vi "PID test.vi"(8 "Enable PID":bool) -> ()   [LabVIEW 2014]
uses:
  PIDstatemachinectl.ctl
  <vilib>/Rock Robotics/WPI/RobotDrive/WPI_RobotDriveGetSetRefNum.vi
panel:
  in  "PID state machine":T1
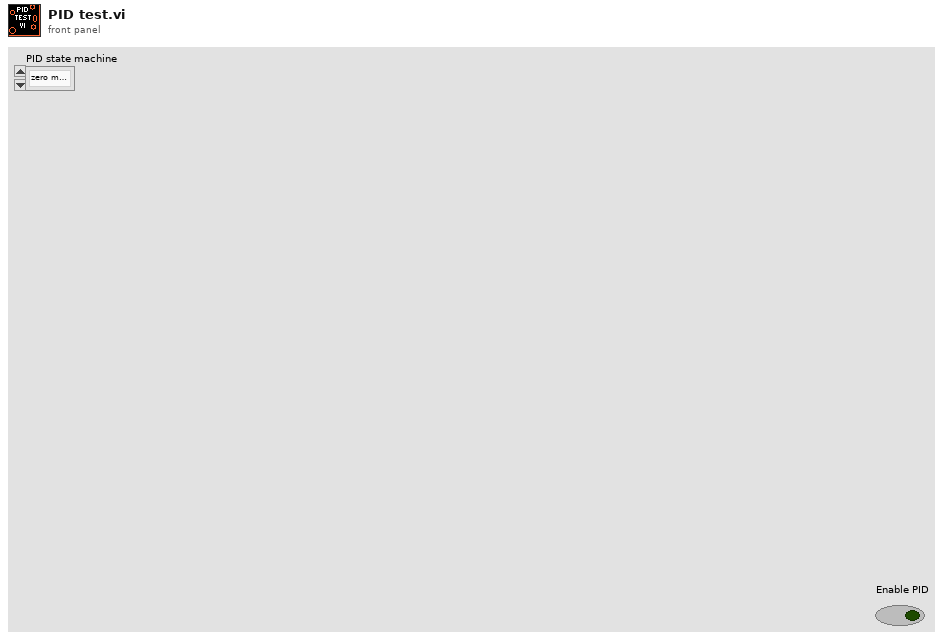
[diagram p1: front panel]
types:
  T1 = typedef "PIDstatemachinectl.ctl" = enum16{"zero motors", "set/run pid", "reset encoder"}
  T2 = typedef "WPI_RobotDriveDevRef.ctl" = cluster{"DevStatus":errorcluster, "Motors[]":T3[], "Square Inputs":bool, "Max Output":dbl}
  T3 = typedef "WPI_MotorControlDeviceRef.ctl" = cluster{"DeviceStatus":errorcluster, "Type":T4, "PWM":cluster{"Controller":T5, "PWM Channel":T6, "DeadBand":T7}, "CAN":cluster{"Device Number":u8, "Control Mode":T8, "Semaphore":T9, "Max Vout":dbl, "TalonSRX Control Mode":T10}, "Invert":bool, "TransformRef":T11, "InvTransformRef":T11}
  T4 = typedef "WPI_MotorControlType.ctl" = enum16{"PWM", "CAN", "CANTalonSRX"}
  T5 = typedef "FPGA_TypedefDigitalModule.ctl" = enum16{"Controller 1"}
  T6 = typedef "FPGA_DIOPWMChannel.ctl" = enum8{"PWM 0", "PWM 1", "PWM 2", "PWM 3", "PWM 4", "PWM 5", "PWM 6", "PWM 7", "PWM 8", "PWM 9", "PWM MXP 0", "PWM MXP 1", "PWM MXP 2", "PWM MXP 3", "PWM MXP 4", "PWM MXP 5", "PWM MXP 6", "PWM MXP 7", "PWM MXP 8", "PWM MXP 9", "Invalid"}
  T7 = typedef "WPI_PWMDeadband.ctl" = cluster{"Name":string, "maxPositivePwm":i32, "minPositivePwm":i32, "centerPwm":i32, "maxNegativePwm":i32, "minNegativePwm":i32, "angularRange":u16}
  T8 = typedef "WPI_CANJaguar_ControlMode.ctl" = enum8{"Percent VBus", "Current", "Speed", "Position", "Voltage"}
  T9 = typedef "Semaphore RefNum" = refnum<k1>
  T10 = typedef "WPI_CANTalonSRX_APIControlMode.ctl" = enum8{"Percent VBus", "Speed", "Position", "Slave", "Unchanged / Invalid"}
  T11 = typedef "WPI_PWMTransform_ConPane.ctl" = refnum<vi>
  T12 = typedef "WPI_EncoderDevRef.ctl" = cluster{"DevStatus":errorcluster, "EncoderIndex":T13, "CounterIndex":T14, "DistancePerCount":dbl, "Decoding Type":T15}
  T13 = typedef "FPGA_EncoderIdx.ctl" = enum8{"Enc 0", "Enc 1", "Enc 2", "Enc 3", "Enc 4", "Enc 5", "Enc 6", "Enc 7", "Invalid"}
  T14 = typedef "FPGA_CounterCtrSystemIndex.ctl" = enum8{"Ctr 0", "Ctr 1", "Ctr 2", "Ctr 3", "Ctr 4", "Ctr 5", "Ctr 6", "Ctr 7", "Invalid"}
  T15 = typedef "WPI_EncoderType.ctl" = enum16{"1x", "2x", "4x"}
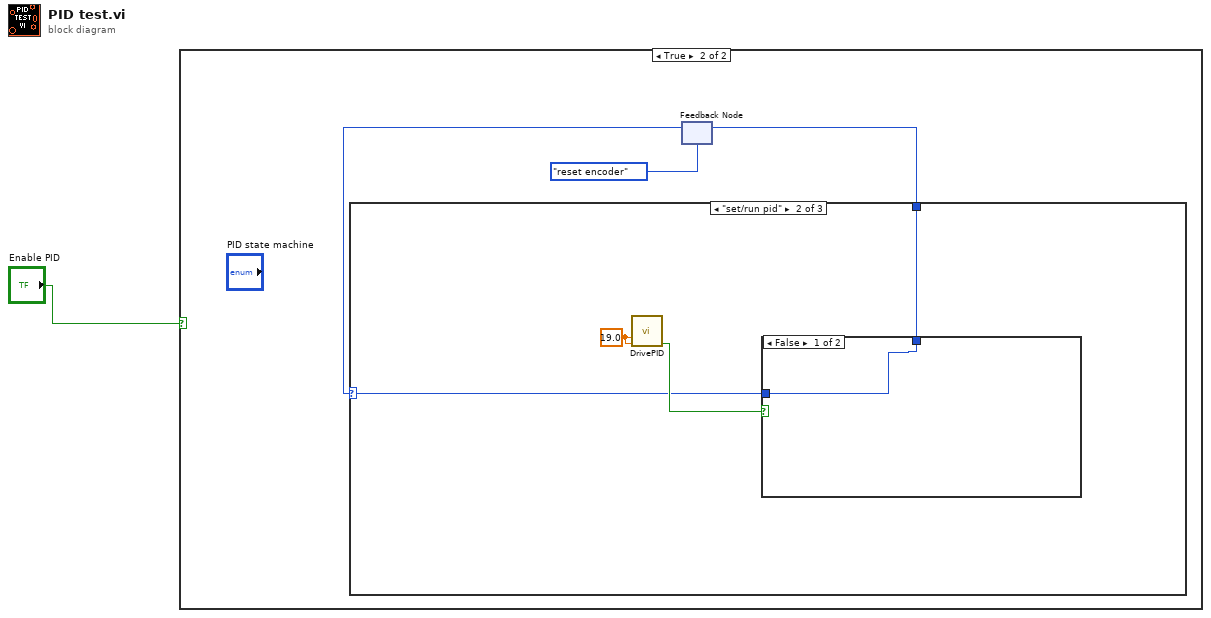
[diagram p0: block diagram]
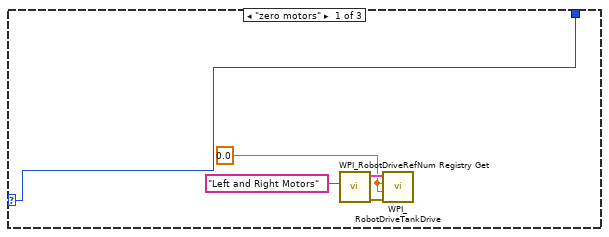
[diagram p3: hidden frame]
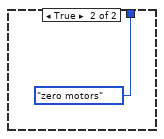
[diagram p4: hidden frame]
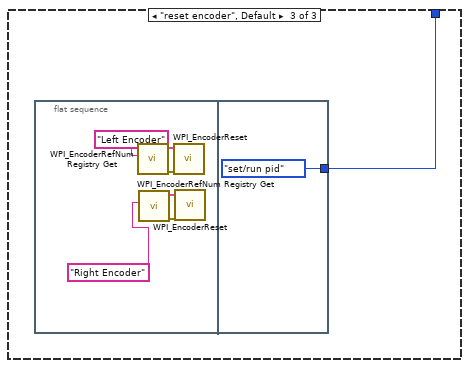
[diagram p5: hidden frame]
diagram:
  n1 = case shown="True" "Enable PID" {
    frame False {
    }
    frame True {
      n2 = feedback #1(PIDstatemachinectl."reset encoder" ("PID state machine")) -> (w3:T1)
      n3 = case shown="\"set/run pid\"" w3 {
        selector: w3 -> [w5 w10 _]
        tunnel: [w5 w11 w16] -> w2
        frame "zero motors" {
          w6 = 0.0 ("Left axis value")
          n4 = call <vilib>:"WPI_RobotDriveRefNum Registry Get.vi"("refnum name"="Left and Right Motors") -> ("error out"=w8:errorcluster, "RobotDriveDevRef"=w7:T2)  [unwired: 9 in]
          n5 = call <vilib>:"WPI_RobotDriveTankDrive.vi"("error in (no error)"=w8, "Right axis value"=w6, "Left axis value"=w6, "RobotDriveDevRef"=w7) -> ()  [unwired: 5 in, 3 out]
        }
        frame "set/run pid" {
          w13 = 19.0 ("SetpointLeft")
          n6 = call "DrivePID.vi"("SetpointLeft"=w13, "SetpointRight"=w13) -> ("Done"=w12:bool)  [unwired: 13 in]
          n7 = case shown="False" w12 {
            tunnel: [w14 PIDstatemachinectl."zero motors" ("PID state machine")] -> w11
            tunnel: w10 -> [w14 _]
            frame False {
            }
            frame True {
            }
          }
        }
        frame "reset encoder", Default {
          n8 = flat-sequence {
            tunnel: [PIDstatemachinectl."set/run pid" ("PID state machine")] -> w16
            frame #0 {
              n9 = call <vilib>:"WPI_EncoderRefNum Registry Get.vi"("refnum name"="Left Encoder") -> ("error out"=w20:errorcluster, "EncoderDevRef"=w19:T12)  [unwired: 9 in]
              n10 = call <vilib>:"WPI_EncoderRefNum Registry Get.vi"("refnum name"="Right Encoder") -> ("error out"=w18:errorcluster, "EncoderDevRef"=w17:T12)  [unwired: 9 in]
              n11 = call <vilib>:"WPI_EncoderReset.vi"("error in (no error)"=w20, "EncoderDevRef"=w19) -> ()  [unwired: 8 in, 2 out]
              n12 = call <vilib>:"WPI_EncoderReset.vi"("error in (no error)"=w18, "EncoderDevRef"=w17) -> ()  [unwired: 8 in, 2 out]
            }
            frame #1 {
            }
          }
        }
      }
      n13 = feedback-in #1(w2) -> ()
    }
  }
